vi "WorkspaceOpenClose.vi"(1 "Open/Close? (T: Open)":bool, 2 "Project Ref in":T1) -> (0 "error out":errorcluster)   [LabVIEW 2015, in "MiscHelperVIs.lvlib"]
uses:
  <vilib>/NI Veristand/Execution/Project/Project Ref.ctl
  NationalInstruments.VeriStand.ClientAPI
  MiscHelperVIs.lvlib
  <vilib>/NI Veristand/Execution/Project/NI_VS Project ExecutionAPI.lvlib
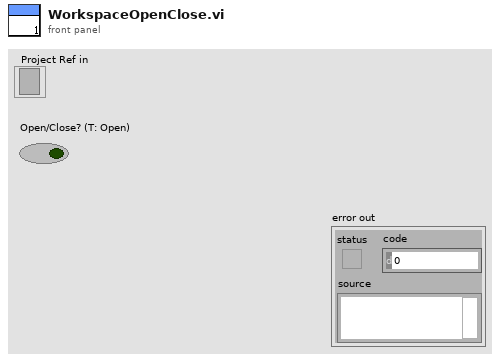
[diagram p1: front panel]
types:
  T1 = typedef "NI_VS Project ExecutionAPI.lvlib/Project Ref.ctl" = refnum<k24>
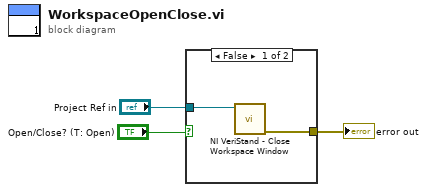
[diagram p0: block diagram]
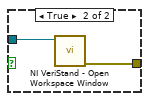
[diagram p2: hidden frame]
diagram:
  n1 = case shown="False" "Open/Close? (T: Open)" {
    tunnel: "Project Ref in" -> [w5 w7]
    tunnel: [w4 w6] -> w2
    frame False {
      n2 = call <vilib>:"NI VeriStand - Close Workspace Window.vi"("Project Ref in"=w5) -> ("error out"=w4:errorcluster)  [unwired: 9 in, 1 out]
    }
    frame True {
      n3 = call <vilib>:"NI VeriStand - Open Workspace Window.vi"("Project Ref in"=w7) -> ("error out"=w6:errorcluster)  [unwired: 9 in, 1 out]
    }
  }
  "error out" <- w2
